vi "cal formulate.vi"(2 "CalData":T1(array[cluster])) -> (6 "caldataout":T1(array[cluster]))   [LabVIEW 2011]
uses:
  <vilib>/express/express arith-compare/Formula/XNode/ExpressFormulaBlockNode.xnode
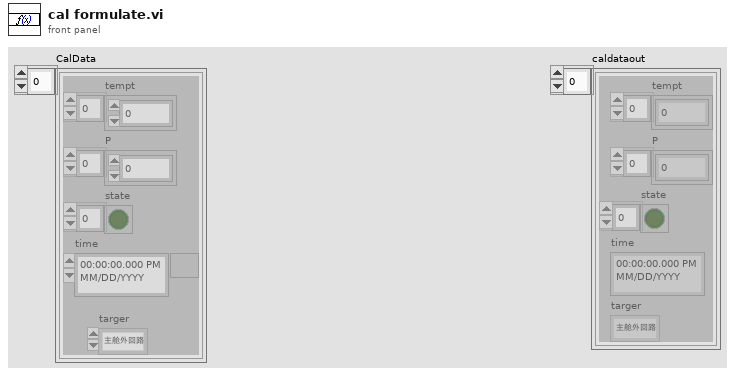
[diagram p1: front panel]
types:
  T1 = cluster{"tempt":dbl[], "P":dbl[], "state":bool[], "time":timestamp, "targer":enum16{"主舱外回路", "主舱内回路", "实验舱外回路", "实验舱内回路"}}[]
  T2 = cluster{"tempt":dbl[], "P":dbl[], "state":bool[], "time":timestamp, "targer":enum16{"主舱外回路", "主舱内回路", "实验舱外回路", "实验舱内回路"}}
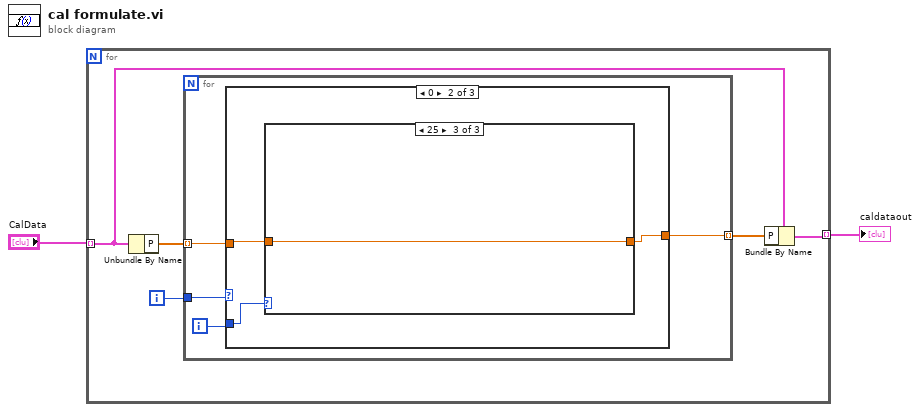
[diagram p0: block diagram]
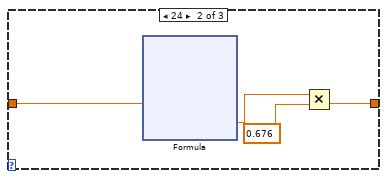
[diagram p4: hidden frame]
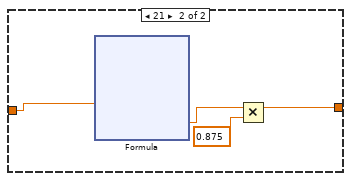
[diagram p6: hidden frame]
diagram:
  n1 = for {
    tunnel: "CalData" -> [w4] mode=indexing
    tunnel: [w3] -> w1 mode=indexing
    i -> [w6]
    n2 = Unbundle By Name(w4) -> ("P"=w7:dbl[])
    n3 = for {
      tunnel: w7 -> [w9] mode=indexing
      tunnel: w6 -> [w10]
      tunnel: [w8] -> w5 mode=indexing
      i -> [w11]
      n4 = case shown="0" w10 {
        tunnel: w11 -> [_ w13 w32]
        tunnel: w9 -> [w12 w15 w31]
        tunnel: [w12 w14 w30] -> w8
        frame 100, Default {
        }
        frame 0 {
          n5 = case shown="25" w13 {
            tunnel: w15 -> [w16 w20 w29]
            tunnel: [w16 w18 w29] -> w14
            frame 100, Default {
            }
            frame 24 {
              n6 = xnode "Formula"("x"=w20) -> ("Result"=w19:dbl)  [unwired: 1 in, 1 out]
              n7 = Multiply(x=w19, y=0.676) -> (x*y=w18:dbl)
            }
            frame 25 {
            }
          }
        }
        frame 1 {
          n8 = case shown="100, Default" w32 {
            tunnel: w31 -> [w33 w37]
            tunnel: [w33 w35] -> w30
            frame 100, Default {
            }
            frame 21 {
              n9 = xnode "Formula"("x"=w37) -> ("Result"=w36:dbl)  [unwired: 1 in, 1 out]
              n10 = Multiply(x=w36, y=0.875) -> (x*y=w35:dbl)
            }
          }
        }
      }
    }
    n11 = Bundle By Name(cluster=w4, "P"=w5) -> (w3:T2)
  }
  "caldataout" <- w1
